vi "ControllerAccumulator.vi"(1 "Input":dbl, 2 "Controller Rate":dbl) -> (0 "Accumulation":dbl)   [LabVIEW 2017]
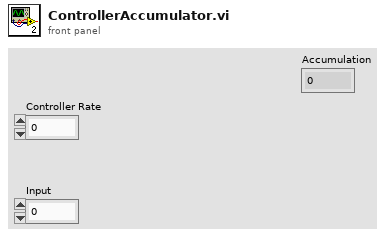
[diagram p1: front panel]
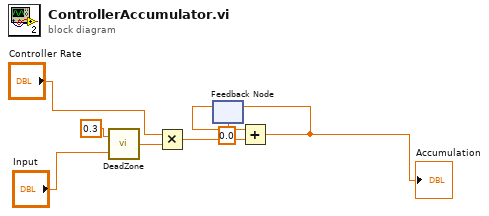
[diagram p0: block diagram]
diagram:
  n1 = call "DeadZone.vi"("Input"="Input", "Tolerance"=0.3) -> ("Output"=w6:dbl)
  n2 = Multiply(x="Controller Rate", y=w6) -> (x*y=w4:dbl)
  n3 = feedback #1(0.0 ("upper limit")) -> (w8:dbl)
  n4 = Add(x=w8, y=w4) -> (x+y=w1:dbl)
  "Accumulation" <- w1
  n5 = feedback-in #1(w1) -> ()
